vi "Two Player Jetpack Working.vi"() -> ()   [LabVIEW 2026]
doc: "Working two player jetpack gameplay loop with stable physics, hazards, scoring, and winner output."
panel:
  out "Final Player 2 Score":dbl
  out "Final Player 1 Score":dbl
  out "Winner Code (1 P1, 2 P2, 0 Draw)":dbl
  out "Game Speed":dbl=1.0
  out "Player 2 Alive":bool=TRUE
  out "Player 1 Alive":bool=TRUE
  out "Player 2 Score":dbl
  out "Player 1 Score":dbl
  out "Player 2 Fuel":dbl=100.0
  out "Player 1 Fuel":dbl=100.0
  out "Player 2 Y":dbl=50.0
  out "Player 1 Y":dbl=50.0
  in  "Player 2 Thrust":bool
  in  "Player 1 Thrust":bool
  in  "Stop":bool
  in  "Player 2 Name":string="Player 2"
  in  "Player 1 Name":string="Player 1"
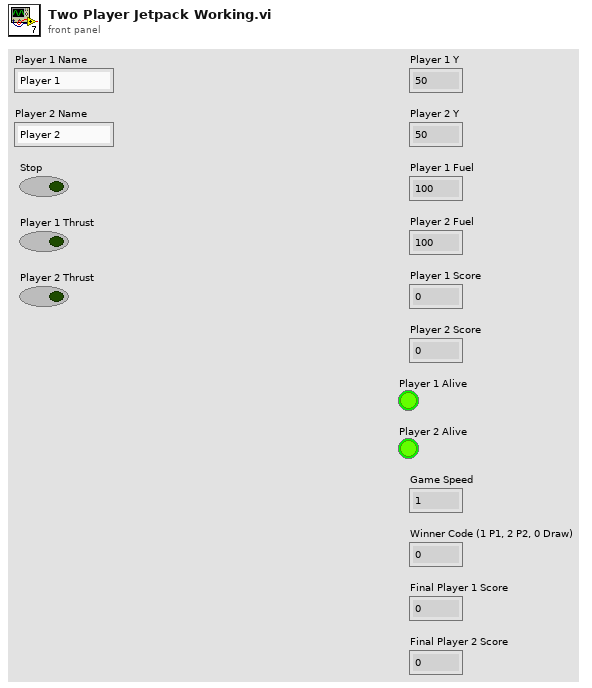
[diagram p1: front panel]
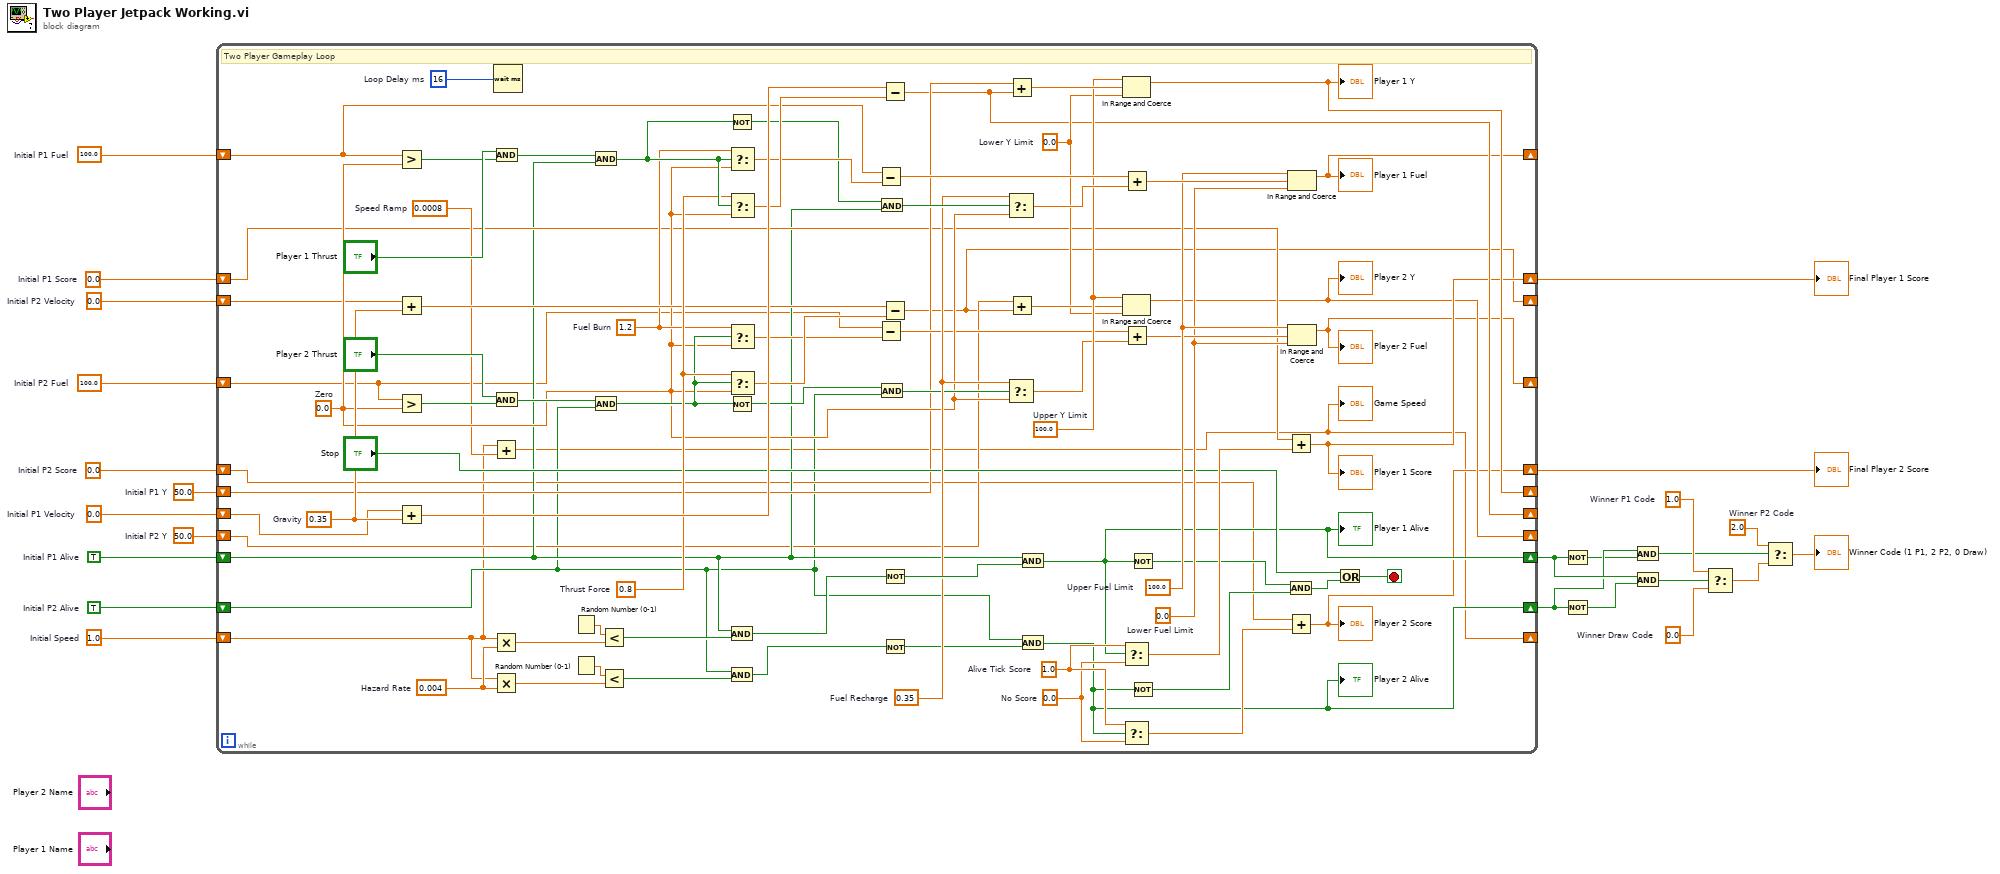
[diagram p0: block diagram]
diagram:
  w6 = 2.0  # Winner P2 Code
  w7 = 0.0  # Winner Draw Code
  w9 = 1.0  # Winner P1 Code
  w14 = 1.0  # Initial Speed
  w15 = TRUE  # Initial P2 Alive
  w16 = 0.0  # Initial P2 Score
  w17 = 100.0  # Initial P2 Fuel
  w18 = 0.0  # Initial P2 Velocity
  w19 = 50.0  # Initial P2 Y
  w20 = TRUE  # Initial P1 Alive
  w21 = 0.0  # Initial P1 Score
  w22 = 100.0  # Initial P1 Fuel
  w23 = 0.0  # Initial P1 Velocity
  w24 = 50.0  # Initial P1 Y
  n1 = while {
    shift-right: [w46] -> _
    shift-left: w24 -> [w45]
    shift-right: [w44] -> _
    shift-left: w23 -> [w43]
    shift-right: [w42] -> _
    shift-left: w22 -> [w41]
    shift-right: [w40] -> w2
    shift-left: w21 -> [w39]
    shift-right: [w38] -> w13
    shift-left: w20 -> [w37]
    shift-right: [w36] -> _
    shift-left: w19 -> [w35]
    shift-right: [w34] -> _
    shift-left: w18 -> [w33]
    shift-right: [w32] -> _
    shift-left: w17 -> [w31]
    shift-right: [w30] -> w1
    shift-left: w16 -> [w29]
    shift-right: [w28] -> w11
    shift-left: w15 -> [w27]
    shift-right: [w26] -> _
    shift-left: w14 -> [w25]
    stop <- w47 stop-if-true
    w52 = u32 16  # Loop Delay ms
    w53 = 0.0008  # Speed Ramp
    w62 = 0.004  # Hazard Rate
    w55 = 0.0  # No Score
    w56 = 1.0  # Alive Tick Score
    w63 = 0.0  # Lower Fuel Limit
    w65 = 100.0  # Upper Fuel Limit
    w70 = 0.35  # Fuel Recharge
    w74 = 1.2  # Fuel Burn
    w75 = 0.0  # Lower Y Limit
    w77 = 100.0  # Upper Y Limit
    w68 = 0.0  # Zero
    w80 = 0.8  # Thrust Force
    w84 = 0.35  # Gravity
    # "Two Player Gameplay Loop"
    n2 = Greater?(x=w41, y=w68) -> (0:w102:bool)
    n3 = Add(x=w33, y=w84) -> (x+y=w79:dbl)
    n4 = Greater?(x=w31, y=w68) -> (0:w82:bool)
    n5 = Add(x=w43, y=w84) -> (x+y=w100:dbl)
    n6 = Add(x=w25, y=w53) -> (x+y=w26:dbl)
    "Game Speed" <- w26
    n7 = Multiply(x=w25, y=w62) -> (x*y=w89:dbl)
    n8 = Multiply(x=w25, y=w62) -> (x*y=w60:dbl)
    n9 = And(x="Player 1 Thrust", y=w102) -> (x .and. y?=w101:bool)
    n10 = And(x="Player 2 Thrust", y=w82) -> (x .and. y?=w81:bool)
    n11 = Wait (ms)(milliseconds to wait=w52) -> ()  [unwired: 1 out]
    n12 = Random Number (0-1)() -> (number: 0 to 1=w90:dbl)
    n13 = Random Number (0-1)() -> (number: 0 to 1=w61:dbl)
    n14 = And(x=w101, y=w37) -> (x .and. y?=w96:bool)
    n15 = And(x=w81, y=w27) -> (x .and. y?=w72:bool)
    n16 = Less?(x=w90, y=w89) -> (x < y?=w88:bool)
    n17 = Less?(x=w61, y=w60) -> (x < y?=w59:bool)
    n18 = Not(x=w96) -> (.not. x?=w95:bool)
    n19 = Not(x=w72) -> (.not. x?=w71:bool)
    n20 = And(x=w37, y=w88) -> (x .and. y?=w87:bool)
    n21 = And(x=w27, y=w59) -> (x .and. y?=w58:bool)
    n22 = Select(t=w74, s=w96, f=w68) -> (s? t:f=w97:dbl)
    n23 = Select(t=w80, s=w96, f=w68) -> (s? t:f=w99:dbl)
    n24 = Select(t=w74, s=w72, f=w68) -> (s? t:f=w73:dbl)
    n25 = Select(t=w80, s=w72, f=w68) -> (s? t:f=w78:dbl)
    n26 = Subtract(x=w41, y=w97) -> (x-y=w93:dbl)
    n27 = Subtract(x=w31, y=w73) -> (x-y=w67:dbl)
    n28 = And(x=w95, y=w37) -> (x .and. y?=w94:bool)
    n29 = And(x=w71, y=w27) -> (x .and. y?=w69:bool)
    n30 = Subtract(x=w100, y=w99) -> (x-y=w44:dbl)
    n31 = Subtract(x=w79, y=w78) -> (x-y=w34:dbl)
    n32 = Not(x=w87) -> (.not. x?=w86:bool)
    n33 = Not(x=w58) -> (.not. x?=w57:bool)
    n34 = Select(t=w70, s=w94, f=w68) -> (s? t:f=w92:dbl)
    n35 = Select(t=w70, s=w69, f=w68) -> (s? t:f=w66:dbl)
    n36 = Add(x=w45, y=w44) -> (x+y=w98:dbl)
    n37 = Add(x=w35, y=w34) -> (x+y=w76:dbl)
    n38 = And(x=w37, y=w86) -> (x .and. y?=w38:bool)
    "Player 1 Alive" <- w38
    n39 = And(x=w27, y=w57) -> (x .and. y?=w28:bool)
    "Player 2 Alive" <- w28
    n40 = In Range and Coerce(upper limit=w77, x=w98, lower limit=w75) -> (coerced(x)=w46:dbl)  [unwired: 1 out]
    "Player 1 Y" <- w46
    n41 = In Range and Coerce(upper limit=w77, x=w76, lower limit=w75) -> (coerced(x)=w36:dbl)  [unwired: 1 out]
    "Player 2 Y" <- w36
    n42 = Select(t=w56, s=w38, f=w55) -> (s? t:f=w85:dbl)
    n43 = Select(t=w56, s=w28, f=w55) -> (s? t:f=w54:dbl)
    n44 = Add(x=w93, y=w92) -> (x+y=w91:dbl)
    n45 = Add(x=w67, y=w66) -> (x+y=w64:dbl)
    n46 = Not(x=w38) -> (.not. x?=w51:bool)
    n47 = Not(x=w28) -> (.not. x?=w50:bool)
    n48 = Add(x=w39, y=w85) -> (x+y=w40:dbl)
    "Player 1 Score" <- w40
    n49 = And(x=w51, y=w50) -> (x .and. y?=w48:bool)
    n50 = Add(x=w29, y=w54) -> (x+y=w30:dbl)
    "Player 2 Score" <- w30
    n51 = In Range and Coerce(upper limit=w65, x=w91, lower limit=w63) -> (coerced(x)=w42:dbl)  [unwired: 1 out]
    "Player 1 Fuel" <- w42
    n52 = In Range and Coerce(upper limit=w65, x=w64, lower limit=w63) -> (coerced(x)=w32:dbl)  [unwired: 1 out]
    "Player 2 Fuel" <- w32
    n53 = Or(x="Stop", y=w48) -> (x .or. y?=w47:bool)
  }
  "Final Player 1 Score" <- w2
  "Final Player 2 Score" <- w1
  n54 = Not(x=w13) -> (.not. x?=w10:bool)
  n55 = Not(x=w11) -> (.not. x?=w12:bool)
  n56 = And(x=w11, y=w10) -> (x .and. y?=w5:bool)
  n57 = And(x=w13, y=w12) -> (x .and. y?=w8:bool)
  n58 = Select(t=w9, s=w8, f=w7) -> (s? t:f=w4:dbl)
  n59 = Select(t=w6, s=w5, f=w4) -> (s? t:f=→"Winner Code (1 P1, 2 P2, 0 Draw)":dbl)
